vi "Query Example.vi"() -> ()   [LabVIEW 2020, in "ORM_Examples.lvlib"]
doc: "Returns the full result set of the query with each row represented by one element of the returned variant array. Note that bbPlayers and BB Players Map classes are not needed for this example."
uses:
  ORM_Examples.lvlib
  194d3a73-cf94-4cc4-bf50-6ab555791e62.vi
  194d3a73-cf94-4cc4-bf50-6ab555791e62.vi/9d007ba8-e96f-4737-8d8a-6b46cf7f5c4a.vi
  194d3a73-cf94-4cc4-bf50-6ab555791e62.vi/050765a8-e5d4-4415-b637-62775228e838.vi
  <vilib>/Viviota/shared/ORM_ADONet.lvlibp/ADOMapper/ADOMapper.lvclass
  C:/Program Files/National Instruments/LabVIEW 2024/vi.lib/Viviota/shared/ORM.lvlibp/ORM/SqlMapper/SqlMapper.lvclass
  <vilib>/Viviota/shared/ORM_DBC_Sqlite.lvlibp/Sqlite Connect.vi
  <vilib>/Utility/error.llb/Error Cluster From Error Code.vi
  <vilib>/Viviota/shared/ORM.lvlibp/ORM/TypeMap/Read TypeMap.vi
  <vilib>/Viviota/shared/ORM.lvlibp/ORM/Query Result/Next.vi
  <vilib>/Viviota/shared/ORM.lvlibp/ORM/TypeMap/ToLabVIEW_Wrap.vi
  <vilib>/Viviota/shared/ORM.lvlibp/ORM/TypeMap/TypeMap.lvclass
  <vilib>/Viviota/shared/ORM.lvlibp/ORM/Query Result/Query Result.lvclass
  ORM_API/ORM_API.lvlib
  <vilib>/Viviota/shared/ORM_ADONet.lvlibp
  <vilib>/Viviota/shared/ORM_DBC_Sqlite.lvlibp/DBC.lvclass
  C:/Program Files/National Instruments/LabVIEW 2024/vi.lib/Viviota/shared/ORM_ADONet.lvlibp/ADOMapper/ADOMapper.lvclass
panel:
  out "Results":variant[](array[variant])
  in  "SQL Query":string
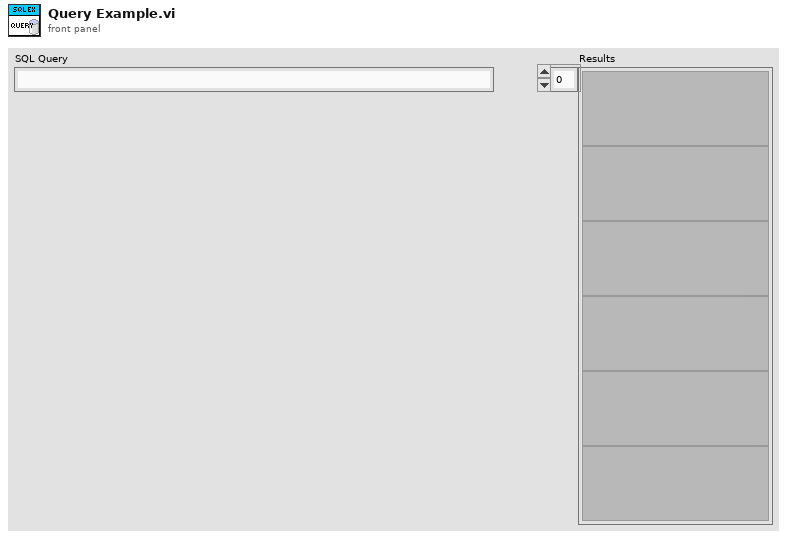
[diagram p1: front panel]
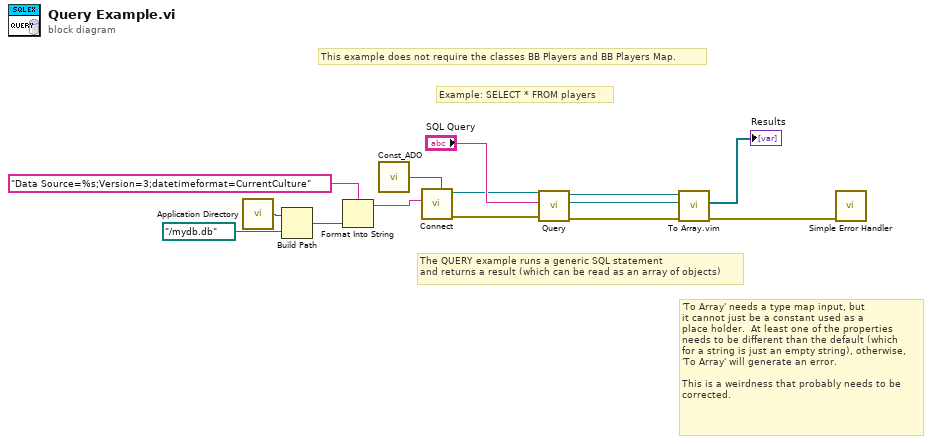
[diagram p0: block diagram]
diagram:
  # "Example: SELECT * FROM players"
  # "The QUERY example runs a generic SQL statement\nand returns a result (which can be read as an array of objects)"
  # "This example does not require the classes BB Players and BB Players Map."
  # "'To Array' needs a type map input, but\nit cannot just be a constant used as a\nplace holder.  At least one of the properties\nneeds to be different than the default (which \nfor a string is just an empty string), otherwise,\n'To Array' will generate an error.\n\nThis is a weirdness that probably needs to be\ncorrected."
  n1 = call <vilib>:"Application Directory.vi"() -> ("Application Directory"=w7:path)
  n2 = Build Path(base path=w7, name or relative path=path "../mydb.db" ("file out")) -> (appended path=w8:path)
  n3 = Format Into String(format string="Data Source=%s;Version=3;datetimeformat=CurrentCulture" ("connectionStringName"), w8) -> (resulting string=w3:string)  [unwired: 2 in, 1 out]
  n4 = call <vilib>:"Const_ADO.vi"() -> ("ADOMapper"=w4:refnum<class "ADOMapper.lvclass">)
  n5 = call-poly "Connect.vi"("SqlMapper Type"=w4, "Connection String"=w3) -> ("error out"=w2:errorcluster, "SqlMapper out"=w1:refnum<class "ADOMapper.lvclass">)  [unwired: 8 in]
  n6 = call-dynamic "Query.vi"("error in (no error)"=w2, "sql"="SQL Query", "ADOMapper in"=w1) -> ("error out"=w14:errorcluster, "Query Result out"=w11:refnum<class "Query Result.lvclass">, "ADOMapper out"=w12:refnum<class "ADOMapper.lvclass">)  [unwired: 6 in]
  n7 = call "To Array.vim"("error in (no error)"=w14, "Query Result in"=w11, "SqlMapper in"=w12) -> ("error out"=w13:errorcluster, "Array"=→"Results":refnum<class>[])  [unwired: 6 in, 1 out]
  n8 = call <vilib>:"Simple Error Handler.vi"("error in (no error)"=w13) -> ()  [unwired: 4 in, 5 out]
